vi "StrikerManMark.vi"(8 "AI Parameters":T1={"GotoKick"={"Dist do cone a frente"=150.0, "attacker farback"=1500.0, "Perto"=300.0, "min dist to kick"=150.0, "kick eps"=0.0, "Time to transition"=0.05}, "Attacker"={"CC chute"=0.09, "CC passe"=0.045, "Kick Force"=100.0, "D ball-robot Kick"=200.0, "D ball-robot Pass"=0.3}, "Defender"={"D max"=1700.0, "Vel p/ robô av"=1000.0, "Kick Force"=100.0, "D atk-def"=0.0, "D farback"=0.0}, "Timeout"={"Field/v in x"=6.0, "Dist Robots"=300, "Dist up in y"=300}, "Pose Striker"={"dist"=200.0, "Numeric"=-4.0, "dist 2"=200.0}, "Dist Stop"=300.0, "Distance when ball out"=200, "D central gap "=150.0, "T pass"=0.0, "Force ++"=0.0, "range kick"=0.0, "Chute alto"=TRUE, "Marcador novo"=TRUE} {"D central gap" format="%#_13g"; "Dist Stop" format="%#_13g"; "Pose Striker"."Numeric" format="%#_13g"; "Defender"."Kick Force" format="%#_13g"; "Defender"."Vel p/ robô av" format="%#_13g"; "Attacker"."D ball-robot Kick" format="%#_13g"; "Attacker"."Kick Force" format="%#_13g"; "Attacker"."CC passe" format="%#_13g"; "Attacker"."CC chute" format="%#_13g"; "GotoKick"."kick eps" format="%#_13g"; "GotoKick"."min dist to kick" format="%#_13g"; "GotoKick"."Perto" format="%#_13g"; "GotoKick"."attacker farback" format="%#_13g"; "GotoKick"."Dist do cone a frente" format="%#_13g"}, 9 "Robot in":T3={"id"=5, "function"=enum."Attacker", "x"=-1842.5054931640625, "y"=520.60986328125, "orientation"=-2.7555055618286133, "v_tangent"=0.0, "v_normal"=0.0, "v_ang"=0.0, "kick_x"=0.0, "kick_z"=0.0, "dribble"=FALSE, "Timestamp"=timestamp(2082758857.4639893 s since 1904-01-01), "dest_x"=0.0, "dest_y"=0.0, "dest_orientation"=0.0, "estimatives"={"est_v_tangent"=0.0, "est_v_normal"=0.0, "est_vx"=0.0, "est_vy"=0.0, "Pos Robot Est"=[]}, "dest_x_kick"=0.0, "dest_y_kick"=0.0, "Gap Coord"=[], "States"=enum."GoToTangent"}, 10 "Field Size in":T7, 11 "IA Input":T2={"our_robots"=[], "enemy_robots"=[], "balls"=[], "geometry"={"line_width"=0, "field_length"=0, "field_width"=0, "boundary_width"=0, "referee_width"=0, "goal_width"=0, "goal_depth"=0, "goal_wall_width"=0, "center_circle_radius"=0, "defense_radius"=0, "defense_stretch"=0, "free_kick_from_defense_dist"=0, "penalty_spot_from_field_line_dist"=0, "penalty_line_from_spot_dist"=0}, "IA Judge"={"stage"="", "command"="", "our_goalie_id"=0.0, "enemy_goalie_id"=0.0, "command enum"=enum."Halt", "Time"=enum."Azul"}, "Received Timestamp"=timestamp(0 s since 1904-01-01), "Events"={"Touch"=FALSE, "Ball out"=FALSE, "id touch"=0.0, "Ball out of \nVision"=FALSE, "Ball inside \nGoalie area"=FALSE, "Robot not responding"=FALSE, "Robots responding status"=[1.0, 1.0, 1.0, 1.0, 1.0, 1.0], "Enemy Ball \nPossession"=FALSE, "Pass State"=FALSE, "id end of pass"=0.0, "Kick"=FALSE, "Id ini Possession"=0.0, "Ball Possesion"=FALSE, "Id Possesion"=0.0}}) -> (2 "Robot out":T3={"id"=0, "function"=enum."Attacker", "x"=0.0, "y"=0.0, "orientation"=0.0, "v_tangent"=0.0, "v_normal"=0.0, "v_ang"=0.0, "kick_x"=0.0, "kick_z"=0.0, "dribble"=FALSE, "Timestamp"=timestamp(0 s since 1904-01-01), "dest_x"=0.0, "dest_y"=0.0, "dest_orientation"=0.0, "estimatives"={"est_v_tangent"=0.0, "est_v_normal"=0.0, "est_vx"=0.0, "est_vy"=0.0, "Pos Robot Est"=[]}, "dest_x_kick"=0.0, "dest_y_kick"=0.0, "Gap Coord"=[], "States"=enum."GoToTangent"}, 3 "id do inimigo\nmais perigoso":u32)   [LabVIEW 2017]
uses:
  Core/Field Size.ctl
  Core/AI Robot.ctl
  Functions Enum.ctl
  AttackerStates.ctl
  Core/AI Input.ctl
  Core/AI Ball.ctl
  Core/AI Judge.ctl
  Command Enum.ctl
  Util/Events/Events.ctl
  AI Parameters.ctl
  <vilib>/Analysis/_algsub.llb/Real Vector Norm.vi
  <vilib>/Analysis/NI_AALPro.lvlib
panel:
  in  "farback striker":dbl=500.0 format="%#_13g"
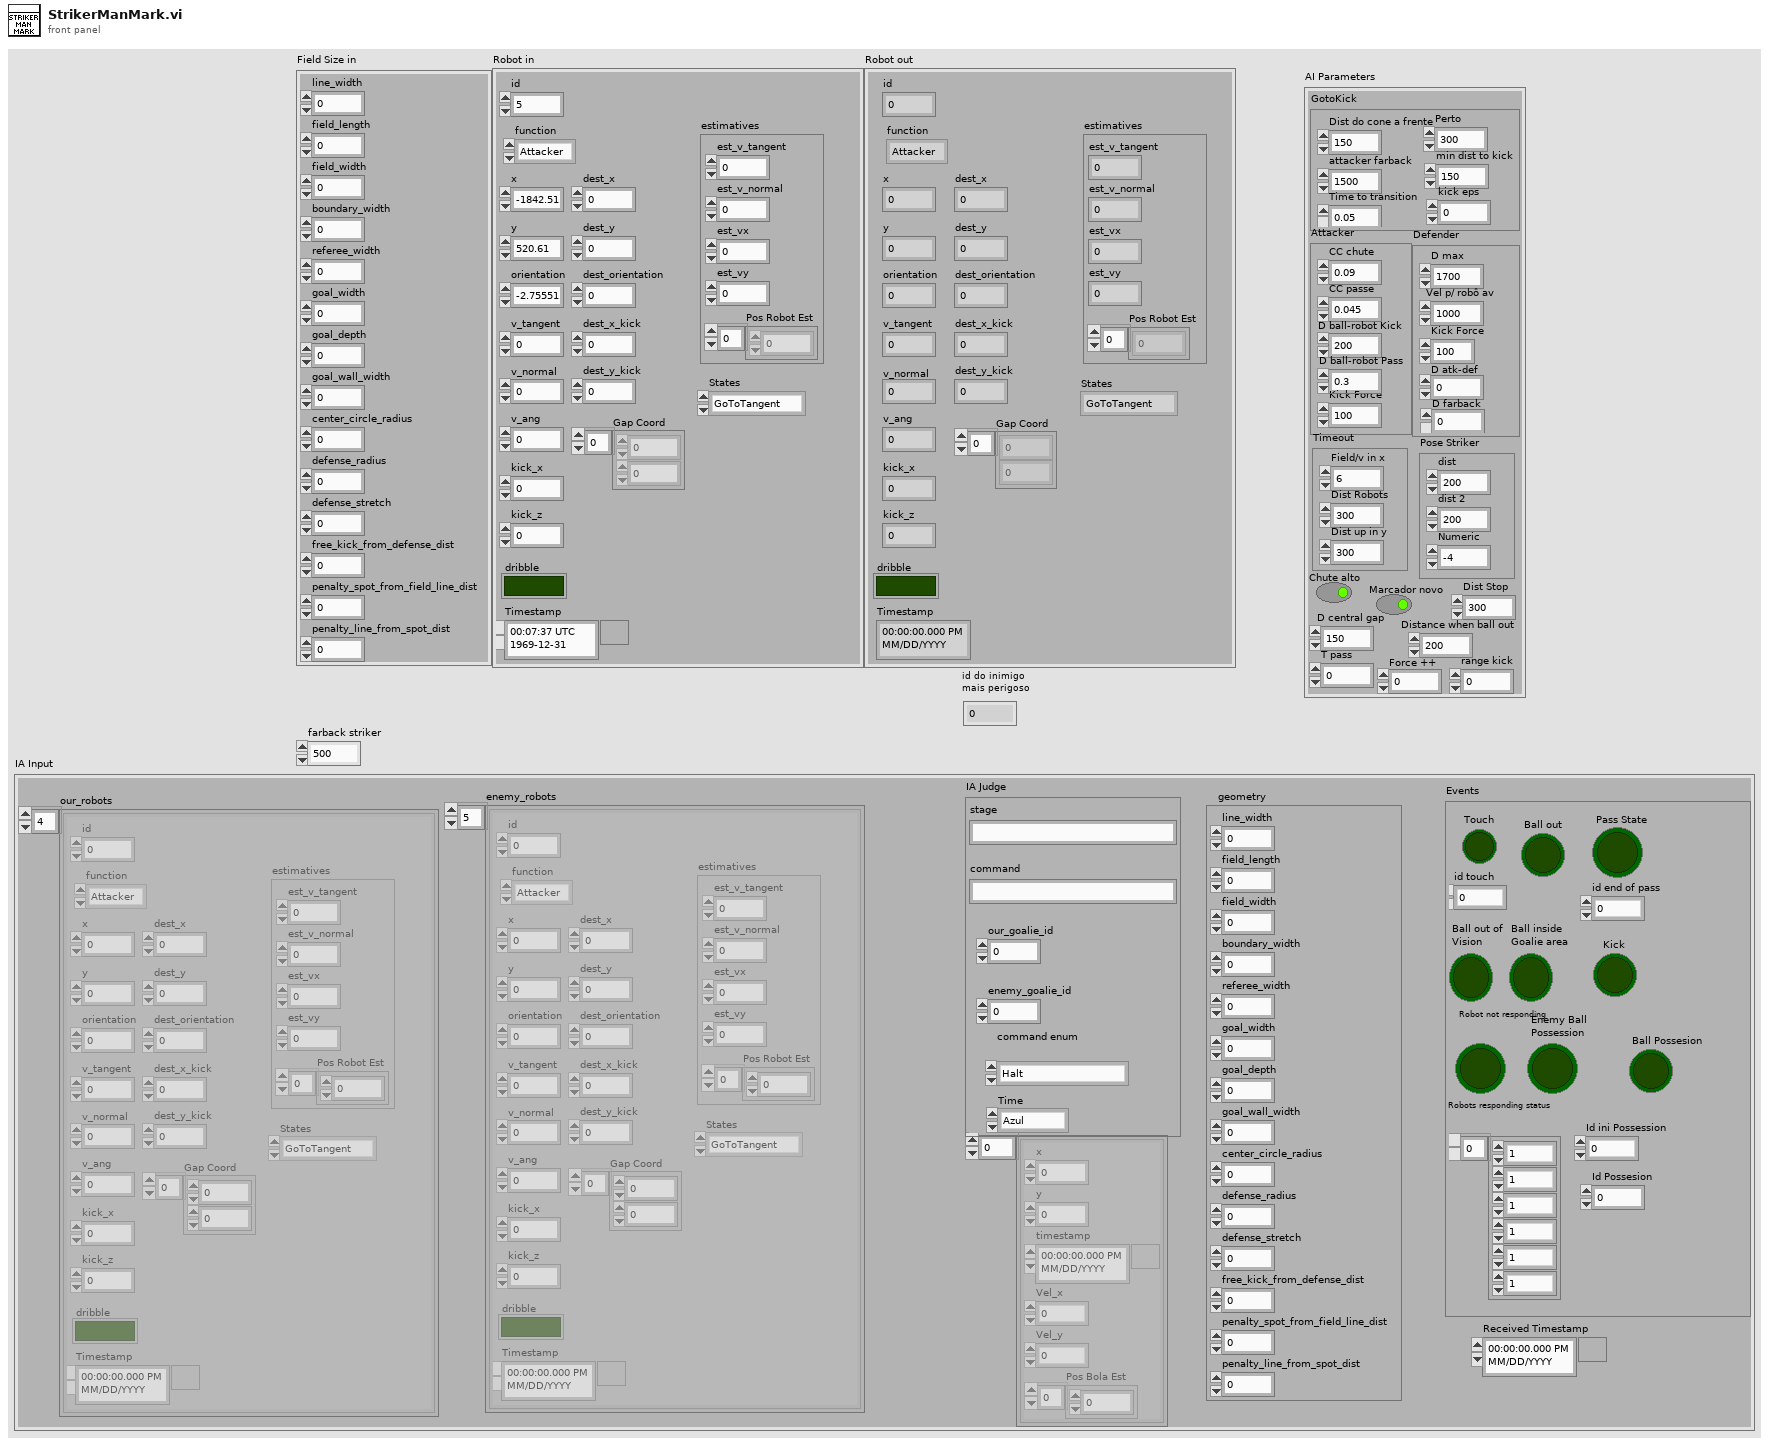
[diagram p1: front panel]
types:
  T1 = typedef "AI Parameters.ctl" = cluster{"GotoKick":cluster{"Dist do cone a frente":dbl, "attacker farback":dbl, "Perto":dbl, "min dist to kick":dbl, "kick eps":dbl, "Time to transition":dbl}, "Attacker":cluster{"CC chute":dbl, "CC passe":dbl, "Kick Force":dbl, "D ball-robot Kick":dbl, "D ball-robot Pass":dbl}, "Defender":cluster{"D max":dbl, "Vel p/ robô av":dbl, "Kick Force":dbl, "D atk-def":dbl, "D farback":dbl}, "Timeout":cluster{"Field/v in x":dbl, "Dist Robots":u32, "Dist up in y":u32}, "Pose Striker":cluster{"dist":dbl, "Numeric":dbl, "dist 2":dbl}, "Dist Stop":dbl, "Distance when ball out":i32, "D central gap ":dbl, "T pass":dbl, "Force ++":dbl, "range kick":dbl, "Chute alto":bool, "Marcador novo":bool}
  T2 = typedef "AI Input.ctl" = cluster{"our_robots":T3[], "enemy_robots":T3[], "balls":T6[], "geometry":T7, "IA Judge":T8, "Received Timestamp":timestamp, "Events":T10}
  T3 = typedef "AI Robot.ctl" = cluster{"id":u32, "function":T4, "x":dbl, "y":dbl, "orientation":dbl, "v_tangent":dbl, "v_normal":dbl, "v_ang":dbl, "kick_x":dbl, "kick_z":dbl, "dribble":bool, "Timestamp":timestamp, "dest_x":dbl, "dest_y":dbl, "dest_orientation":dbl, "estimatives":cluster{"est_v_tangent":dbl, "est_v_normal":dbl, "est_vx":dbl, "est_vy":dbl, "Pos Robot Est":dbl[]}, "dest_x_kick":dbl, "dest_y_kick":dbl, "Gap Coord":dbl[], "States":T5}
  T4 = typedef "Functions Enum.ctl" = enum16{"Attacker", "Goalie", "Defender", "Striker", "Goto 0", "Dummy", "Kicker", "ZigZag"}
  T5 = typedef "AttackerStates.ctl" = enum16{"Pass", "GoToTangent", "BallGetting", "GoToKick", ""}
  T6 = typedef "AI Ball.ctl" = cluster{"x":dbl, "y":dbl, "timestamp":timestamp, "Vel_x":dbl, "Vel_y":dbl, "Pos Bola Est":dbl[]}
  T7 = typedef "Field Size.ctl" = cluster{"line_width":u32, "field_length":u32, "field_width":u32, "boundary_width":u32, "referee_width":u32, "goal_width":u32, "goal_depth":u32, "goal_wall_width":u32, "center_circle_radius":u32, "defense_radius":u32, "defense_stretch":u32, "free_kick_from_defense_dist":u32, "penalty_spot_from_field_line_dist":u32, "penalty_line_from_spot_dist":u32}
  T8 = typedef "AI Judge.ctl" = cluster{"stage":string, "command":string, "our_goalie_id":dbl, "enemy_goalie_id":dbl, "command enum":T9, "Time":enum16{"Azul", "Amarelo"}}
  T9 = typedef "Command Enum.ctl" = enum16{"Halt", "Stop", "Force Start", "PKA Normal Start", "Prepare Kickoff Ally", "PKE Normal Start", "Prepare Kickoff Enemy", "Prepare Penalty Ally", "PPA Normal Start", "Prepare Penalty Enemy", "PPE Normal Start", "Direct Free Enemy", "Direct Free Ally", "Indirect Free Enemy", "Indirect Free Ally", "Timeout Enemy", "Timeout Ally", "Goal Enemy", "Goal Ally", "Ball Placement Enemy", "Ball Placement Ally", "Normal Half Time", "Extra Time Break", "Extra Half Time", "None", "Post Game"}
  T10 = typedef "Events.ctl" = cluster{"Touch":bool, "Ball out":bool, "id touch":dbl, "Ball out of \nVision":bool, "Ball inside \nGoalie area":bool, "Robot not responding":bool, "Robots responding status":dbl[], "Enemy Ball \nPossession":bool, "Pass State":bool, "id end of pass":dbl, "Kick":bool, "Id ini Possession":dbl, "Ball Possesion":bool, "Id Possesion":dbl}
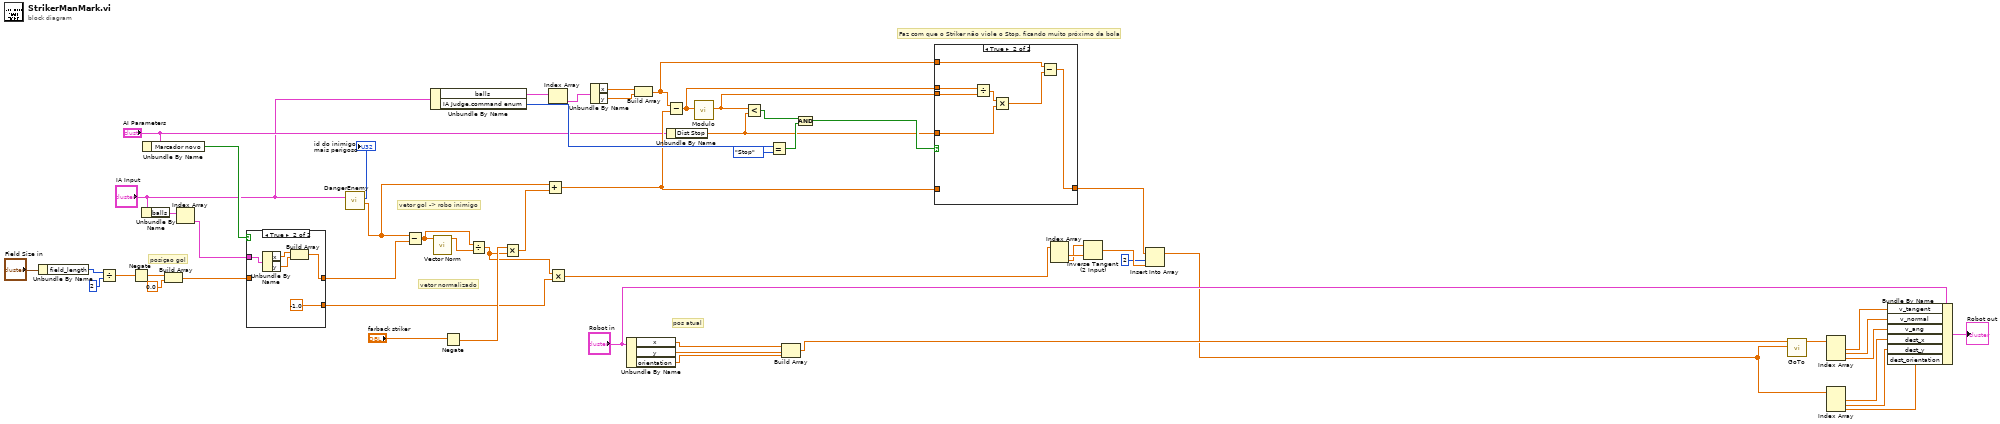
[diagram p0: block diagram]
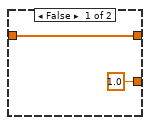
[diagram p2: hidden frame]
diagram:
  # "Faz com que o Striker não viole o Stop, ficando muito próximo da bola"
  # "pos atual"
  # "vetor normalizado"
  # "vetor gol -> robo inimigo"
  # "posiçao gol"
  n1 = Unbundle By Name("Field Size in") -> ("field_length"=w55:u32)
  n2 = Divide(x=w55, y=u32 2) -> (x/y=w53:dbl)
  n3 = Negate(x=w53) -> (-x=w52:dbl)
  n4 = Unbundle By Name("IA Input") -> ("balls"=w7:T6[])
  n5 = Unbundle By Name("AI Parameters") -> ("Marcador novo"=w9:bool)
  n6 = Build Array(w52, 0.0 ("element")) -> (w12:dbl[])
  n7 = Index Array(array=w7) -> (element=w6:T6)  [unwired: 1 in]
  n8 = case shown="True" w9 {
    tunnel: [w58 w60] -> w11
    tunnel: w12 -> [w58 _]
    tunnel: w6 -> [_ w63]
    tunnel: [1.0 -1.0] -> w1
    frame False {
    }
    frame True {
      n9 = Unbundle By Name(w63) -> ("x"=w62:dbl, "y"=w61:dbl)
      n10 = Build Array(w62, w61) -> (w60:dbl[])
    }
  }
  n11 = call "DangerEnemy.vi"("IA Input"="IA Input") -> ("Pos do inimigo\nperigoso"=w31:dbl[], "id do inimigo\nmais perigoso"=→"id do inimigo\nmais perigoso":u32)  [unwired: 9 in]
  n12 = Subtract(x=w31, y=w11) -> (x-y=w49:dbl[])
  n13 = Unbundle By Name("IA Input") -> ("balls"=w26:T6[], "IA Judge.command enum"=w20:T9)
  n14 = call-poly <vilib>:"Vector Norm.vi"("Input Vector"=w49) -> ("norm"=w50:dbl)  [unwired: 9 in, 1 out]
  n15 = Negate(x="farback striker") -> (-x=w29:dbl)
  n16 = Divide(x=w49, y=w50) -> (x/y=w3:dbl[])
  n17 = Multiply(x=w29, y=w3) -> (x*y=w28:dbl[])
  n18 = Add(x=w31, y=w28) -> (x+y=w17:dbl[])
  n19 = Index Array(array=w26) -> (element=w25:T6)  [unwired: 1 in]
  n20 = Multiply(x=w3, y=w1) -> (x*y=w2:dbl[])
  n21 = Unbundle By Name(w25) -> ("x"=w24:dbl, "y"=w23:dbl)
  n22 = Unbundle By Name("Robot in") -> ("x"=w44:dbl, "y"=w43:dbl, "orientation"=w42:dbl)
  n23 = Build Array(w24, w23) -> (w14:dbl[])
  n24 = Unbundle By Name("AI Parameters") -> ("Dist Stop"=w15:dbl)
  n25 = Subtract(x=w14, y=w17) -> (x-y=w13:dbl[])
  n26 = call "Modulo.vi"("2D vector"=w13) -> ("Modulo"=w16:dbl)  [unwired: 10 in]
  n27 = Less?(x=w16, y=w15) -> (x < y?=w22:bool)
  n28 = Equal?(x=w20, y=Command_Enum."Stop") -> (x = y?=w21:bool)
  n29 = Build Array(w44, w43, w42) -> (w41:dbl[])
  n30 = And(x=w22, y=w21) -> (x .and. y?=w18:bool)
  n31 = case shown="True" w18 {
    tunnel: [w64 w66] -> w5
    tunnel: w17 -> [w64 _]
    tunnel: w16 -> [_ w71]
    tunnel: w15 -> [_ w69]
    tunnel: w14 -> [_ w68]
    tunnel: w13 -> [_ w65]
    frame False {
    }
    frame True {
      n32 = Divide(x=w65, y=w71) -> (x/y=w70:dbl[])
      n33 = Multiply(x=w70, y=w69) -> (x*y=w67:dbl[])
      n34 = Subtract(x=w68, y=w67) -> (x-y=w66:dbl[])
    }
  }
  n35 = Index Array(array=w2) -> (element #1=w48:dbl, element #2=w47:dbl)  [unwired: 2 in]
  n36 = Inverse Tangent (2 Input)(1:w48, 2:w47) -> (0:w46:dbl)
  n37 = Insert Into Array(array=w5, index=2, new element=w46) -> (w4:dbl[])
  n38 = call "GoTo.vi"("Target"=w4, "Position"=w41) -> ("Output\nVelocity"=w40:dbl[])  [unwired: 8 in, 1 out]
  n39 = Index Array(array=w40) -> (element #1=w39:dbl, element #2=w38:dbl, element #3=w37:dbl)  [unwired: 3 in]
  n40 = Index Array(array=w4) -> (element #1=w36:dbl, element #2=w35:dbl, element #3=w34:dbl)  [unwired: 3 in]
  n41 = Bundle By Name(cluster="Robot in", "v_tangent"=w39, "v_normal"=w38, "v_ang"=w37, "dest_x"=w36, "dest_y"=w35, "dest_orientation"=w34) -> (→"Robot out":T3)
